vi "SQL_CreateTables.vi"(9 "SubAssembly":string, 10 "LineName":string, 11 "ConnectionDSN":string) -> ()   [LabVIEW 2017]
panel:
  in  "CreateTables":bool
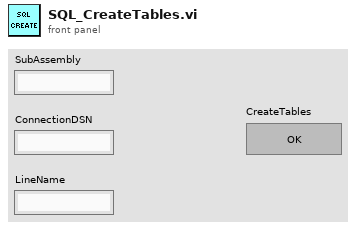
[diagram p1: front panel]
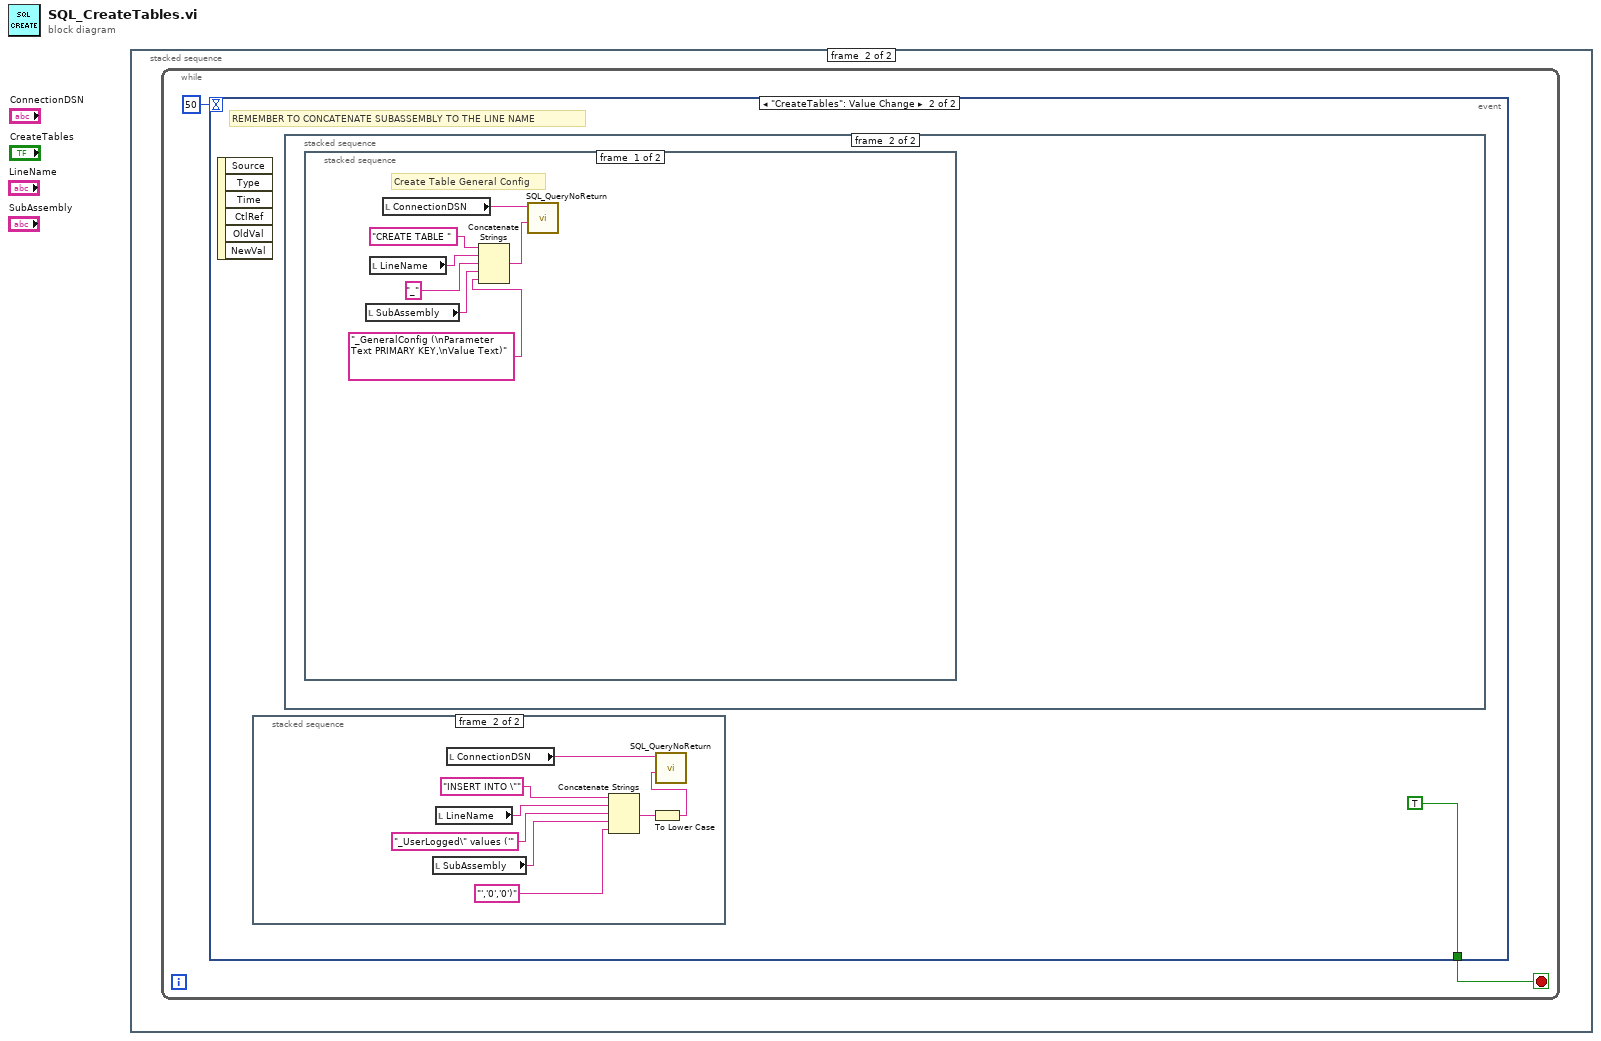
[diagram p0: block diagram]
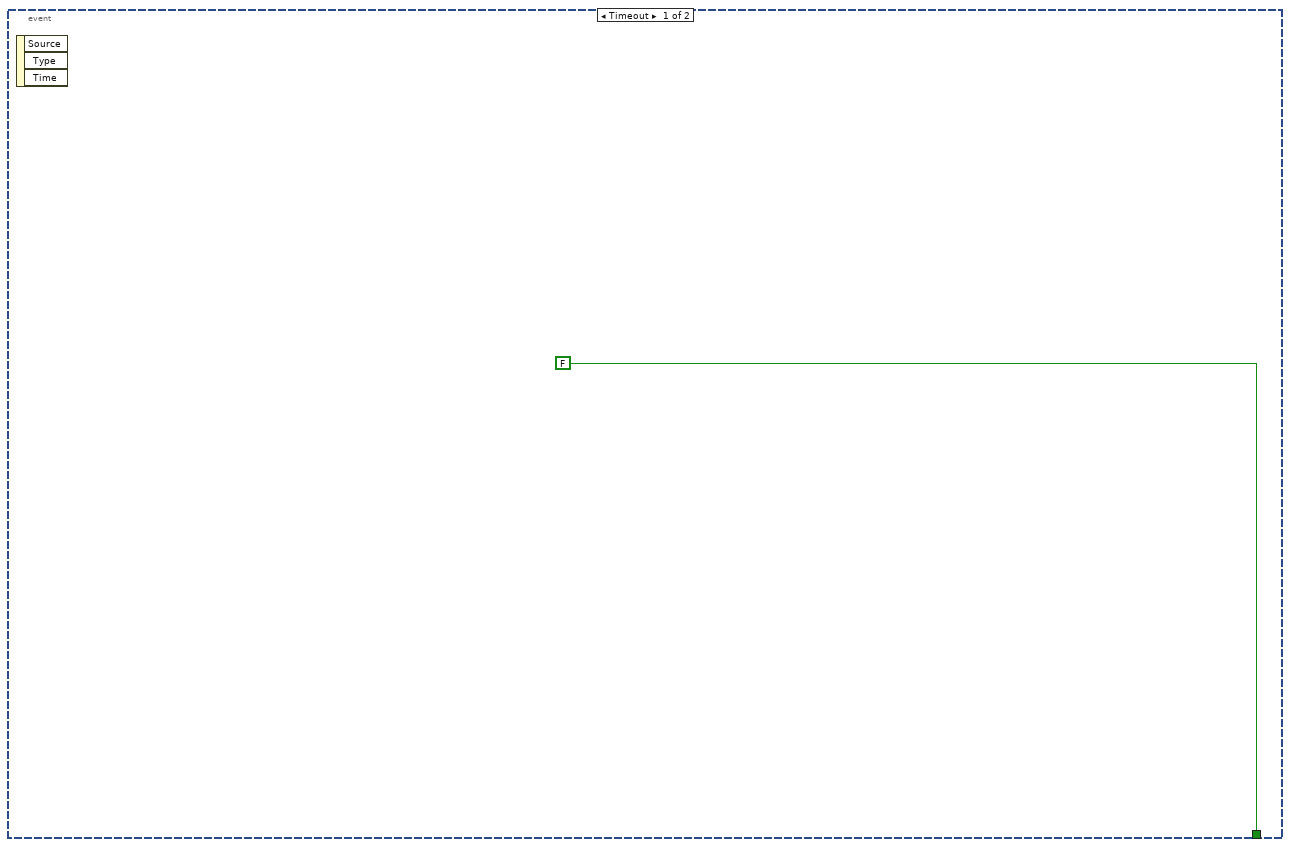
[diagram p3: hidden frame]
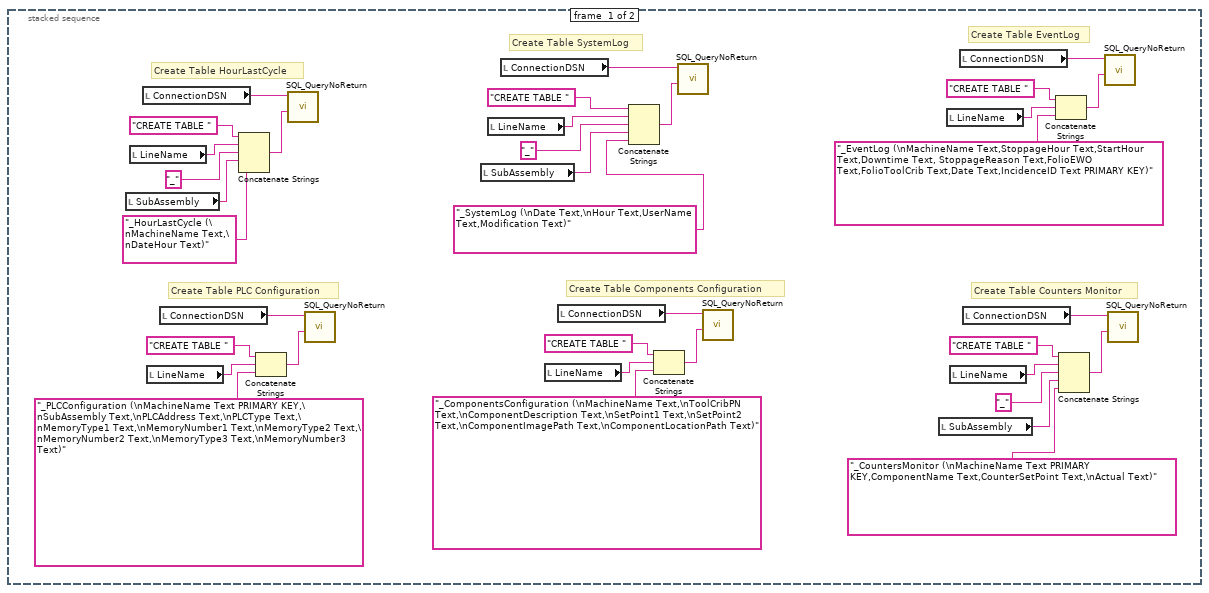
[diagram p4: hidden frame]
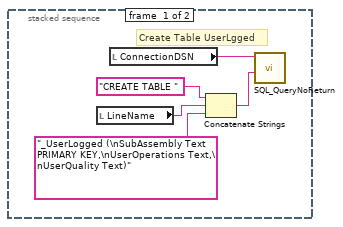
[diagram p6: hidden frame]
diagram:
  n1 = stacked-sequence {
    frame #0 {
    }
    frame #1 {
      n2 = while {
        stop <- w1 stop-if-true
        n3 = event shown="[1] \"CreateTables\": Value Change" {
          selector: _ -> [_ _]
          dyn-events: _ -> [_ _]
          timeout: 50 -> [_ _]
          tunnel: [FALSE TRUE] -> w1
          event Timeout {
            n4 = event-data() -> ()  [unwired: 1 in, 3 out]
          }
          event "CreateTables": Value Change {
            # "REMEMBER TO CONCATENATE SUBASSEMBLY TO THE LINE NAME"
            n5 = event-data() -> ()  [unwired: 1 in, 6 out]
            n6 = stacked-sequence {
              frame #0 {
                # "Create Table UserLgged"
                n7 = local read "LineName"() -> (w50:string)
                n8 = local read "ConnectionDSN"() -> (w48:string)
                n9 = Concatenate Strings("CREATE TABLE " ("SQL query"), w50, "_UserLogged (\nSubAssembly Text PRIMARY KEY,\nUserOperations Text,\nUserQuality Text)" ("SQL query")) -> (w52:string)
                n10 = call "SQL_QueryNoReturn.vi"("SQL query"=w52, "ConnectionDSN"=w48) -> ()  [unwired: 10 in]
              }
              frame #1 {
                n11 = local read "SubAssembly"() -> (w60:string)
                n12 = local read "LineName"() -> (w59:string)
                n13 = local read "ConnectionDSN"() -> (w58:string)
                n14 = Concatenate Strings("INSERT INTO \"" ("SQL query"), w59, "_UserLogged\" values ('" ("SQL query"), w60, "','0','0')" ("SQL query")) -> (w54:string)
                n15 = To Lower Case(string=w54) -> (all lower case string=w53:string)
                n16 = call "SQL_QueryNoReturn.vi"("SQL query"=w53, "ConnectionDSN"=w58) -> ()  [unwired: 10 in]
              }
            }
            n17 = stacked-sequence {
              frame #0 {
                # "Create Table Counters Monitor"
                # "Create Table Components Configuration"
                # "Create Table PLC Configuration"
                # "Create Table EventLog"
                # "Create Table SystemLog"
                # "Create Table HourLastCycle"
                n18 = local read "SubAssembly"() -> (w6:string)
                n19 = local read "LineName"() -> (w38:string)
                n20 = local read "ConnectionDSN"() -> (w40:string)
                n21 = local read "LineName"() -> (w25:string)
                n22 = local read "ConnectionDSN"() -> (w23:string)
                n23 = Concatenate Strings("CREATE TABLE " ("SQL query"), w38, "_", w6, "_HourLastCycle (\nMachineName Text,\nDateHour Text)" ("SQL query")) -> (w37:string)
                n24 = Concatenate Strings("CREATE TABLE " ("SQL query"), w25, "_PLCConfiguration (\nMachineName Text PRIMARY KEY,\nSubAssembly Text,\nPLCAddress Text,\nPLCType Text,\nMemoryType1 Text,\nMemoryNumber1 Text,\nMemoryType2 Text,\nMemoryNumber2 Text,\nMemoryType3 Text,\nMemoryNumber3 Text)" ("SQL query")) -> (w27:string)
                n25 = call "SQL_QueryNoReturn.vi"("SQL query"=w37, "ConnectionDSN"=w40) -> ()  [unwired: 10 in]
                n26 = call "SQL_QueryNoReturn.vi"("SQL query"=w27, "ConnectionDSN"=w23) -> ()  [unwired: 10 in]
                n27 = local read "SubAssembly"() -> (w9:string)
                n28 = local read "LineName"() -> (w35:string)
                n29 = local read "ConnectionDSN"() -> (w33:string)
                n30 = local read "LineName"() -> (w20:string)
                n31 = local read "ConnectionDSN"() -> (w22:string)
                n32 = Concatenate Strings("CREATE TABLE " ("SQL query"), w35, "_", w9, "_SystemLog (\nDate Text,\nHour Text,UserName Text,Modification Text)" ("SQL query")) -> (w36:string)
                n33 = Concatenate Strings("CREATE TABLE " ("SQL query"), w20, "_ComponentsConfiguration (\nMachineName Text,\nToolCribPN Text,\nComponentDescription Text,\nSetPoint1 Text,\nSetPoint2 Text,\nComponentImagePath Text,\nComponentLocationPath Text)" ("SQL query")) -> (w18:string)
                n34 = call "SQL_QueryNoReturn.vi"("SQL query"=w36, "ConnectionDSN"=w33) -> ()  [unwired: 10 in]
                n35 = call "SQL_QueryNoReturn.vi"("SQL query"=w18, "ConnectionDSN"=w22) -> ()  [unwired: 10 in]
                n36 = local read "SubAssembly"() -> (w12:string)
                n37 = local read "LineName"() -> (w30:string)
                n38 = local read "LineName"() -> (w16:string)
                n39 = local read "ConnectionDSN"() -> (w32:string)
                n40 = local read "ConnectionDSN"() -> (w14:string)
                n41 = Concatenate Strings("CREATE TABLE " ("SQL query"), w30, "_EventLog (\nMachineName Text,StoppageHour Text,StartHour Text,Downtime Text, StoppageReason Text,FolioEWO Text,FolioToolCrib Text,Date Text,IncidenceID Text PRIMARY KEY)" ("SQL query")) -> (w28:string)
                n42 = Concatenate Strings("CREATE TABLE " ("SQL query"), w16, "_" ("SQL query"), w12, "_CountersMonitor (\nMachineName Text PRIMARY KEY,ComponentName Text,CounterSetPoint Text,\nActual Text)" ("SQL query")) -> (w17:string)
                n43 = call "SQL_QueryNoReturn.vi"("SQL query"=w28, "ConnectionDSN"=w32) -> ()  [unwired: 10 in]
                n44 = call "SQL_QueryNoReturn.vi"("SQL query"=w17, "ConnectionDSN"=w14) -> ()  [unwired: 10 in]
              }
              frame #1 {
                n45 = stacked-sequence {
                  frame #0 {
                    # "Create Table General Config"
                    n46 = local read "SubAssembly"() -> (w44:string)
                    n47 = local read "LineName"() -> (w46:string)
                    n48 = local read "ConnectionDSN"() -> (w47:string)
                    n49 = Concatenate Strings("CREATE TABLE " ("SQL query"), w46, "_", w44, "_GeneralConfig (\nParameter Text PRIMARY KEY,\nValue Text)" ("SQL query")) -> (w45:string)
                    n50 = call "SQL_QueryNoReturn.vi"("SQL query"=w45, "ConnectionDSN"=w47) -> ()  [unwired: 10 in]
                  }
                  frame #1 {
                  }
                }
              }
            }
          }
        }
      }
    }
  }
